vi "Find Multiple Added Highlight.vi"(11 "Test Case In":refnum<class "Find Hughlights Test.lvclass">) -> (0 "error out":errorcluster, 3 "Test Case Out":refnum<class "Find Hughlights Test.lvclass">)   [LabVIEW 2020, in "Find Hughlights Test.lvclass"]
uses:
  Find Hughlights Test.lvclass
  C:/Program Files (x86)/National Instruments/LabVIEW 2020/vi.lib/Astemes/LUnit/Test Case.lvclass
  <vilib>/Astemes/LUnit/Test Case.lvclass/Test Case.ctl
  4993e8ee-a06a-463a-9684-69129f64d5ce.vi
  <vilib>/Astemes/LUnit/Append Pass Result.vi
  <vilib>/Astemes/LUnit/Append Fail Result.vi
  <vilib>/Astemes/LUnit/Describe Comparison.vi
  4993e8ee-a06a-463a-9684-69129f64d5ce.vi/9c5d11cd-9439-4240-a1ee-d9baace9c924.vi
  <vilib>/Astemes/LUnit/Run In UI.vi
  <vilib>/Utility/error.llb/Clear Errors.vi
  <vilib>/Astemes/LUnit/Describe Variant.vi
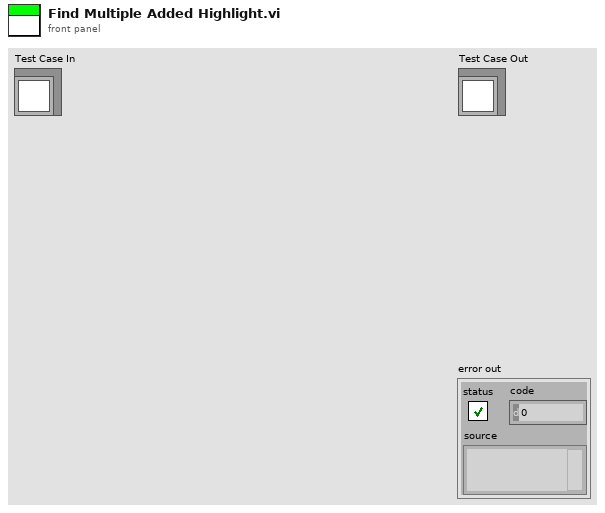
[diagram p1: front panel]
types:
  T1 = cluster{"Selection Start":u32, "Selection End":u32}
  T2 = cluster{"Selection Start":u32, "Selection End":u32}[]
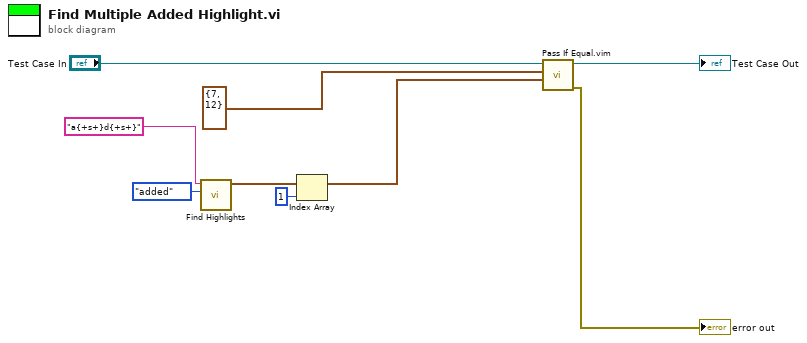
[diagram p0: block diagram]
diagram:
  n1 = call "Find Highlights.vi"("Type"=enum16{"added", "missing"}."added", "String"="a{+s+}d{+s+}" ("Reference")) -> ("Sections"=w4:T2)  [unwired: 9 in]
  n2 = Index Array(array=w4, index=1) -> (element=w2:T1)
  n3 = call "Pass If Equal.vim"("Actual"=w2, "Expected"=T1 {"Selection Start"=7, "Selection End"=12}, "LUnit Test Case In"="Test Case In") -> ("error out"=→"error out":errorcluster, "LUnit Test Case Out"=→"Test Case Out":refnum<class "Find Hughlights Test.lvclass">)  [unwired: 7 in]
